vi "Configure Horizontal Timing.vi"(0 "Scope Reference":refnum<k15>, 5 "Minimum Sampling Rate (S/s)":dbl format="%#_6p", 7 "Record Length":i32 min=0 max=100, 11 "error in":errorcluster) -> (4 "Scope Reference Out":refnum<k15>, 15 "error out":errorcluster)   [LabVIEW 2020, in "LDO PSRR.lvlib"]
uses:
  LDO PSRR.lvlib
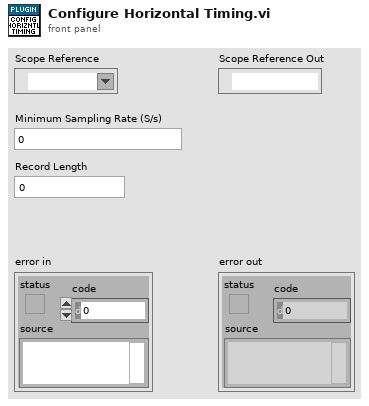
[diagram p1: front panel]
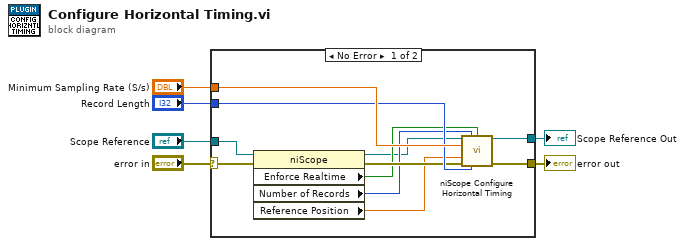
[diagram p0: block diagram]
diagram:
  n1 = case shown="No Error" "error in" {
    selector: "error in" -> [w15 w19]
    tunnel: "Minimum Sampling Rate (S/s)" -> [w17 _]
    tunnel: "Record Length" -> [w16 _]
    tunnel: [w14 w19] -> w3
    tunnel: "Scope Reference" -> [w12 w18]
    tunnel: [w7 w18] -> w1
    frame No Error {
      n2 = property class="niScope"(reference=w12, error in=w15) -> (reference out=w8:refnum<k15>, error out=w13:errorcluster, "Enforce Realtime"=w11:bool, "Number of Records"=w10:i32, "Reference Position"=w9:dbl)
      n3 = call <instrlib>:"niScope Configure Horizontal Timing.vi"("instrument handle"=w8, "number of records"=w10, "enforce realtime"=w11, "min sample rate"=w17, "reference position"=w9, "error in"=w13, "min record length"=w16) -> ("instrument handle out"=w7:refnum<k15>, "error out"=w14:errorcluster)  [unwired: 7 in]
    }
    frame Error {
    }
  }
  "error out" <- w3
  "Scope Reference Out" <- w1
